vi "SaveChoice_Paper1(SubVI).vi"(7 "RanFilenames":string[](array[string]), 8 "Previous 2":refnum<vi>, 9 "Next 2":refnum<vi>, 10 "connection reference":T1, 11 "Array":refnum<vi>[](array[refnum])) -> ()   [LabVIEW 2013]
uses:
  <vilib>/addons/database/Connection.llb/Conn ObjectReference.ctl
  FYP_LabviewGlobal(SubVI).vi
  <vilib>/addons/database/NI_Database_API.lvlib
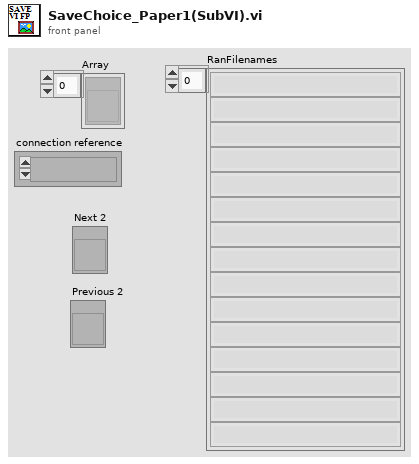
[diagram p1: front panel]
types:
  T1 = typedef "NI_Database_API.lvlib/Conn ObjectReference.ctl" = refnum<k1>
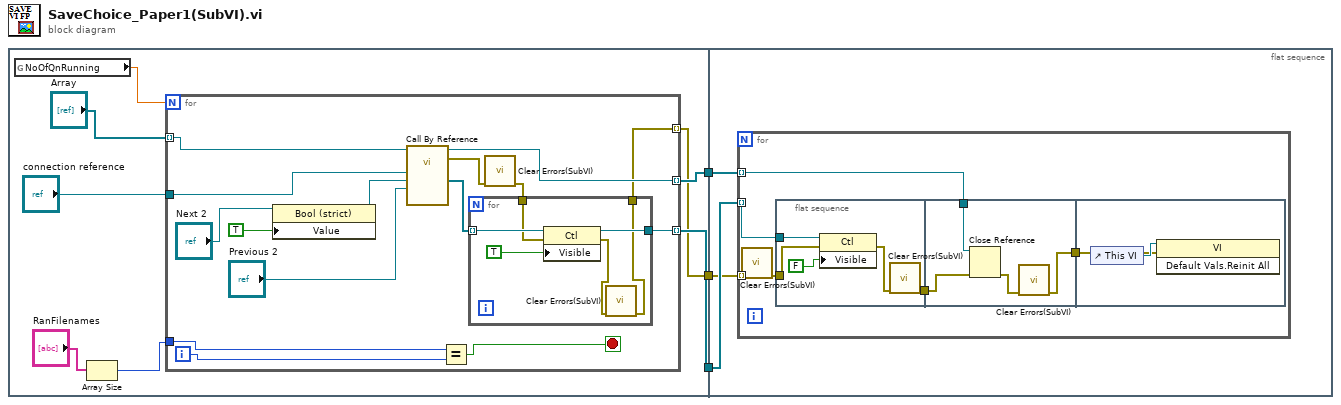
[diagram p0: block diagram]
diagram:
  n1 = flat-sequence {
    tunnel: [w8] -> w3
    tunnel: [w7] -> w2
    tunnel: [w4] -> w1
    tunnel: w3 -> [w34]
    tunnel: w2 -> [w35]
    tunnel: w1 -> [w33]
    frame #0 {
      n2 = global read "FYP_LabviewGlobal(SubVI).vi" "NoOfQnRunning"() -> (w5:dbl)
      n3 = Array Size(array="RanFilenames") -> (size(s)=w6:i32)
      n4 = for {
        N: w5 -> [_]
        tunnel: "Array" -> [w23] mode=indexing
        tunnel: "connection reference" -> [w21]
        tunnel: [w22] -> w7 mode=indexing
        tunnel: [w24] -> w8 mode=indexing
        tunnel: w6 -> [w17]
        tunnel: [w12] -> w4 mode=indexing
        i -> [w15]
        stop <- w16 stop-if-true
        n5 = property class="Bool (strict)"(reference="Next 2", "Value"=TRUE) -> (reference out=w20:refnum<vi>)  [unwired: 1 in, 1 out]
        n6 = call-by-ref "?"(reference=w23, "Previous 2"="Previous 2", "Next 2"=w20, "connection reference"=w21) -> (reference out=w22:refnum<vi>, error out=w14:errorcluster, "Array"=w18:refnum<vi>[])  [unwired: 9 in]
        n7 = Equal?(x=w17, y=w15) -> (x = y?=w16:bool)
        n8 = call "Clear Errors(SubVI).vi"("error in (no error)"=w14) -> ("error out"=w13:errorcluster)  [unwired: 6 in]
        n9 = for {
          tunnel: w18 -> [w32] mode=indexing
          tunnel: [w30] -> w24
          tunnel: w13 -> [w29]
          tunnel: [w27] -> w12
          n10 = property class="Ctl"(reference=w32, error in=w29, "Visible"=TRUE) -> (reference out=w30:refnum<vi>, error out=w28:errorcluster)
          n11 = call "Clear Errors(SubVI).vi"("error in (no error)"=w28) -> ("error out"=w27:errorcluster)  [unwired: 6 in]
        }
      }
    }
    frame #1 {
      n12 = for {
        tunnel: w35 -> [w40] mode=indexing
        tunnel: w34 -> [w41] mode=indexing
        tunnel: w33 -> [w39] mode=indexing
        n13 = call "Clear Errors(SubVI).vi"("error in (no error)"=w39) -> ("error out"=w38:errorcluster)  [unwired: 6 in]
        n14 = flat-sequence {
          tunnel: w41 -> [w46]
          tunnel: w38 -> [w44]
          tunnel: [w42] -> w36
          tunnel: w40 -> [w50]
          tunnel: [w47] -> w37
          tunnel: w36 -> [w49]
          tunnel: w37 -> [w51]
          frame #0 {
            n15 = property class="Ctl"(reference=w46, error in=w44, "Visible"=FALSE) -> (error out=w43:errorcluster)  [unwired: 1 out]
            n16 = call "Clear Errors(SubVI).vi"("error in (no error)"=w43) -> ("error out"=w42:errorcluster)  [unwired: 6 in]
          }
          frame #1 {
            n17 = Close Reference(reference=w50, error in (no error)=w49) -> (error out=w48:errorcluster)
            n18 = call "Clear Errors(SubVI).vi"("error in (no error)"=w48) -> ("error out"=w47:errorcluster)  [unwired: 6 in]
          }
          frame #2 {
            n19 = control-ref of="This VI"() -> (w52:refnum<vi>)
            n20 = invoke class="VI" method="Default Vals.Reinit All"(reference=w52, error in=w51) -> ()  [unwired: 1 in, 3 out]
          }
        }
      }
    }
  }
